vi "Example 12 - Modifying Typedefs.vi"() -> ()   [LabVIEW 2015]
uses:
  source/Scripting.lvlib
panel:
  in  "Enum":enum16{"String", "Number", "Boolean", "Cluster"}(ring)
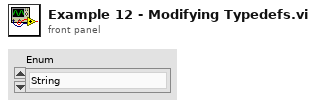
[diagram p1: front panel]
types:
  T1 = cluster{"Number":i32, "String":string, "Boolean":bool}
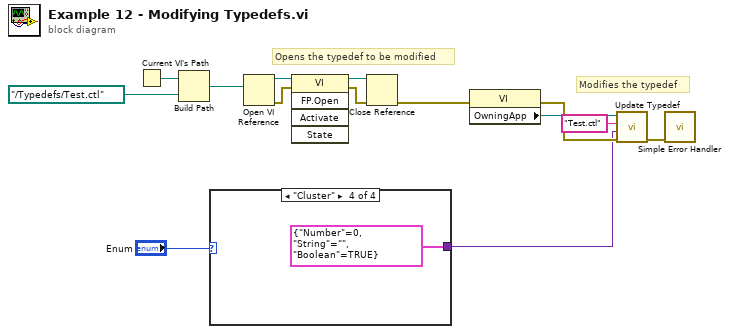
[diagram p0: block diagram]
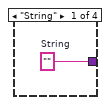
[diagram p2: hidden frame]
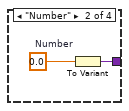
[diagram p3: hidden frame]
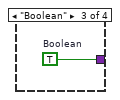
[diagram p4: hidden frame]
diagram:
  # "Modifies the typedef"
  # "Opens the typedef to be modified"
  n1 = Current VI's Path() -> (path=w14:path)
  n2 = Build Path(base path=w14, name or relative path=path "../Typedefs/Test.ctl") -> (appended path=w12:path)
  n3 = case shown="\"Cluster\"" "Enum" {
    tunnel: [w15 w16 w18 T1 {"Number"=0, "String"="", "Boolean"=TRUE}] -> w1
    frame "String" {
      w15 = ""  # String
    }
    frame "Number" {
      w17 = 0.0  # Number
      n4 = To Variant(anything=w17) -> (Variant=w16:variant)
    }
    frame "Boolean" {
      w18 = TRUE  # Boolean
    }
    frame "Cluster" {
    }
  }
  n5 = Open VI Reference(vi path=w12) -> (vi reference=w11:refnum<vi>, error out=w10:errorcluster)  [unwired: 5 in]
  n6 = invoke class="VI" method="FP.Open"(reference=w11, error in=w10) -> (reference out=w8:refnum<vi>, error out=w9:errorcluster)  [unwired: 3 in, 3 out]
  n7 = Close Reference(reference=w8, error in (no error)=w9) -> (error out=w6:errorcluster)
  n8 = property class="VI"(error in=w6) -> (error out=w5:errorcluster, "OwningApp"=w7:refnum<vi>)  [unwired: 1 in, 1 out]
  n9 = call "Update Typedef.vi"("error in (no error)"=w5, "Data Type"=w1, "Name"="Test.ctl", "Application in"=w7) -> ("error out"=w2:errorcluster)  [unwired: 4 in, 3 out]
  n10 = call <vilib>:"Simple Error Handler.vi"("error in (no error)"=w2) -> ()  [unwired: 4 in, 5 out]
